vi "Ex2_PRINCIPAL(SM).vi"() -> ()   [LabVIEW 2020]
uses:
  <vilib>/MakerHub/LINX/LMH-LINX.lvlib
panel:
  in  "Serial Port":refnum<visa-resource-name>="COM4"
  in  "stop":bool
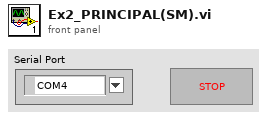
[diagram p1: front panel]
types:
  T1 = enum16{"Configura", "Adquiere", "Procesa", "Grafica y Guarda", "Termina"}
  T2 = typedef "LMH-LINX.lvlib/LINX Ref.ctl" = cluster{"IO":T3, "Interface":T4, "LINX Device Config":T5}
  T3 = typedef "LMH-LINX.lvlib/Platform.ctl" = enum16{"Remote", "Local"}
  T4 = typedef "LMH-LINX.lvlib/Interface.ctl" = enum16{"Serial", "TCP"}
  T5 = typedef "LMH-LINX.lvlib/Device.lvlib/LINX Device Config.ctl" = cluster{"Interface":T4, "COM Port":refnum<visa-resource-name>, "TCP Configuration":T6, "Device Family":u8, "Device ID":u8, "Device Name":string, "TCP Ref":refnum<k5>, "Channels":T7}
  T6 = typedef "LMH-LINX.lvlib/Device.lvlib/TCP Config.ctl" = cluster{"IP Address":string, "Port":u16}
  T7 = typedef "LMH-LINX.lvlib/Channels.ctl" = cluster{"DI":u8[], "DO":u8[], "AI":u8[], "AO":u8[], "PWM":u8[], "QE":u8[], "UART":u8[], "I2C 2":u8[], "SPI":u8[], "CAN":u8[], "Servo":u8[], "AI Ref (V)":dbl, "AI Resolution (Bits)":u8, "AO Ref (V)":dbl, "AO Resolution (Bits)":u8}
  T8 = cluster{"Temp":dbl, "Volt":dbl, "Humd":dbl, "Ant":bool, "Ctrl":bool, "ErrCtr":bool, "Aceler":dbl, "Boolean":bool}
  T9 = cluster{"Ant":bool, "ErrCtr":bool, "Volt":dbl, "Humd":dbl, "Aceler":dbl, "Ctrl":bool, "Sts_Tx-Rx":bool, "Temp":dbl}
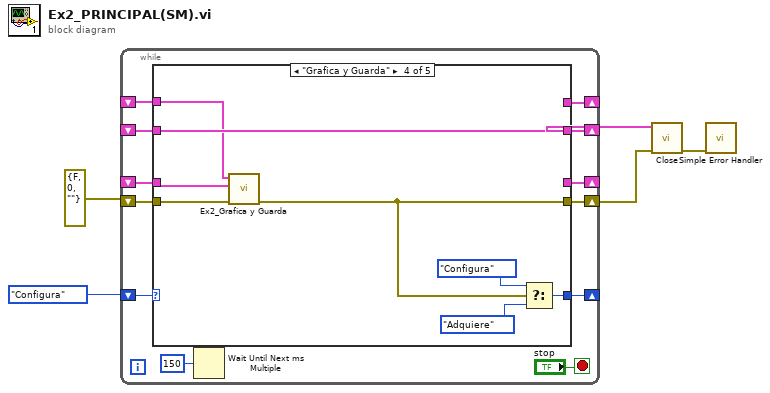
[diagram p0: block diagram]
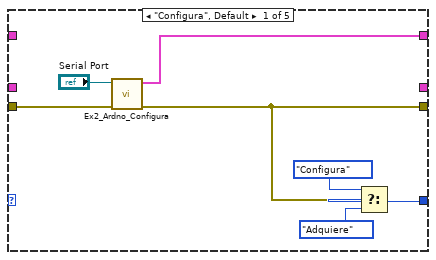
[diagram p2: hidden frame]
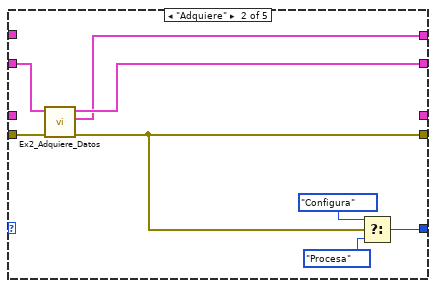
[diagram p3: hidden frame]
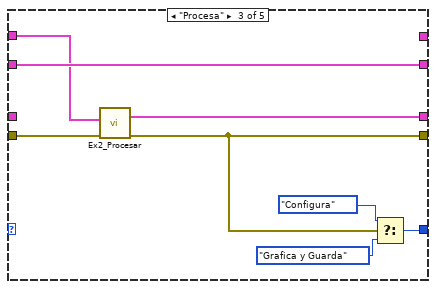
[diagram p4: hidden frame]
diagram:
  n1 = while {
    shift-right: [w17] -> w4
    shift-left: _ -> [w13]
    shift-right: [w16] -> w5
    shift-left: errorcluster {"status"=FALSE, "code"=0, "source"=""} ("error constant") -> [w14]
    shift-right: [w15] -> _
    shift-left: T1."Configura" -> [w9]
    shift-right: [w12] -> _
    shift-left: _ -> [w11]
    shift-right: [w7] -> _
    shift-left: _ -> [w6]
    stop <- "stop" stop-if-true
    n2 = case shown="\"Grafica y Guarda\"" w9 {
      tunnel: [w20 w29 w35 w48 w50] -> w17
      tunnel: [w19 w30 w36 w42 w49] -> w16
      tunnel: [w21 w31 w38 w44 _] -> w15
      tunnel: w14 -> [w22 w32 w37 w47 w49]
      tunnel: w13 -> [_ w27 w35 w48 w50]
      tunnel: [_ w28 _ _ w51] -> w12
      tunnel: w11 -> [_ _ w34 w41 w51]
      tunnel: [_ _ w33 _ _] -> w7
      tunnel: w6 -> [_ _ _ w43 _]
      frame "Configura", Default {
        n3 = call "Ex2_Ardno_Configura.vi"("Error In"=w22, "Serial Port"="Serial Port") -> ("Error Out"=w19:errorcluster, "LINX Resource"=w20:T2)  [unwired: 8 in]
        n4 = Select(t=T1."Configura", s=w19, f=T1."Adquiere") -> (s? t:f=w21:T1)
      }
      frame "Adquiere" {
        n5 = call "Ex2_Adquiere_Datos.vi"("error in (no error)"=w32, "LINX Resource in"=w27) -> ("error out"=w30:errorcluster, "Señales"=w28:T8, "LINX Resource out"=w29:T2)  [unwired: 7 in]
        n6 = Select(t=T1."Configura", s=w30, f=T1."Procesa") -> (s? t:f=w31:T1)
      }
      frame "Procesa" {
        n7 = call "Ex2_Procesar.vi"("error in (no error)"=w37, "Señales"=w34) -> ("error out"=w36:errorcluster, "Señales Procesadas"=w33:T9)  [unwired: 8 in]
        n8 = Select(t=T1."Configura", s=w36, f=T1."Grafica y Guarda") -> (s? t:f=w38:T1)
      }
      frame "Grafica y Guarda" {
        n9 = call "Ex2_Grafica y Guarda.vi"("error in (no error)"=w47, "Señales Procesadas"=w43, "Señales"=w41) -> ("error out"=w42:errorcluster)  [unwired: 6 in, 2 out]
        n10 = Select(t=T1."Configura", s=w42, f=T1."Adquiere") -> (s? t:f=w44:T1)
      }
      frame "Termina" {
      }
    }
    n11 = Wait Until Next ms Multiple(millisecond multiple=u32 150) -> ()  [unwired: 1 out]
  }
  n12 = call <vilib>:"Close.vi"("Error In"=w5, "LINX Resource"=w4) -> ("Error Out"=w1:errorcluster)  [unwired: 9 in]
  n13 = call <vilib>:"Simple Error Handler.vi"("error in (no error)"=w1) -> ()  [unwired: 4 in, 5 out]
